vi "SignExtensiontab.vi"(2 "Input Bits":dbl=18.0, 3 "inputs":u32[](array[numeric]) format="%x") -> (0 "scalarOutput":i32, 1 "outputs":i32[](array[numeric]))   [LabVIEW 2014]
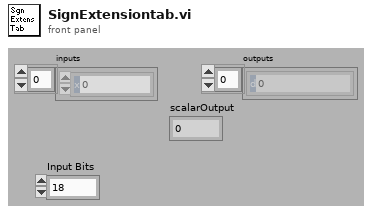
[diagram p1: front panel]
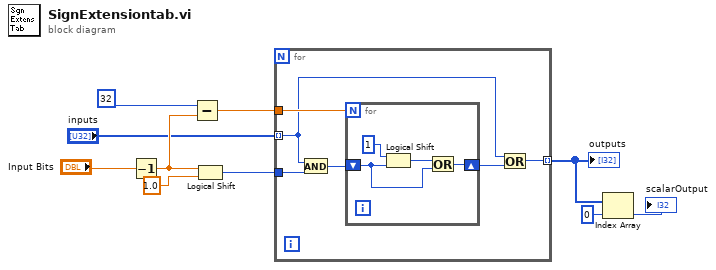
[diagram p0: block diagram]
diagram:
  n1 = Decrement(x="Input Bits") -> (x-1=w5:dbl)
  n2 = Subtract(x=32 ("Input Bits"), y=w5) -> (x-y=w8:dbl)
  n3 = Logical Shift(y=w5, x=1.0) -> (x << y=w9:u32)
  n4 = for {
    tunnel: w9 -> [w16]
    tunnel: w8 -> [w15]
    tunnel: "inputs" -> [w12] mode=indexing
    tunnel: [w11] -> w3 mode=indexing
    n5 = And(x=w12, y=w16) -> (x .and. y?=w14:u32)
    n6 = for {
      N: w15 -> [_]
      shift-right: [w17] -> w13
      shift-left: w14 -> [w18]
      n7 = Logical Shift(y=u32 1 ("x"), x=w18) -> (x << y=w19:u32)
      n8 = Or(x=w19, y=w18) -> (x .or. y?=w17:u32)
    }
    n9 = Or(x=w12, y=w13) -> (x .or. y?=w11:u32)
  }
  "outputs" <- w3
  n10 = Index Array(array=w3, index=0) -> (element=→"scalarOutput":u32)
